vi "File_name_to_number.vi"(10 "Folder Path":path) -> (0 "Base File Name":string, 1 "Last file number":i32, 2 "File number =  file name?":bool, 3 "All Files in Dir":path[](array[path]))   [LabVIEW 2016]
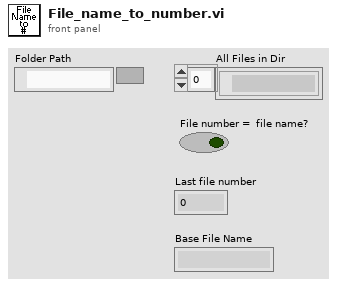
[diagram p1: front panel]
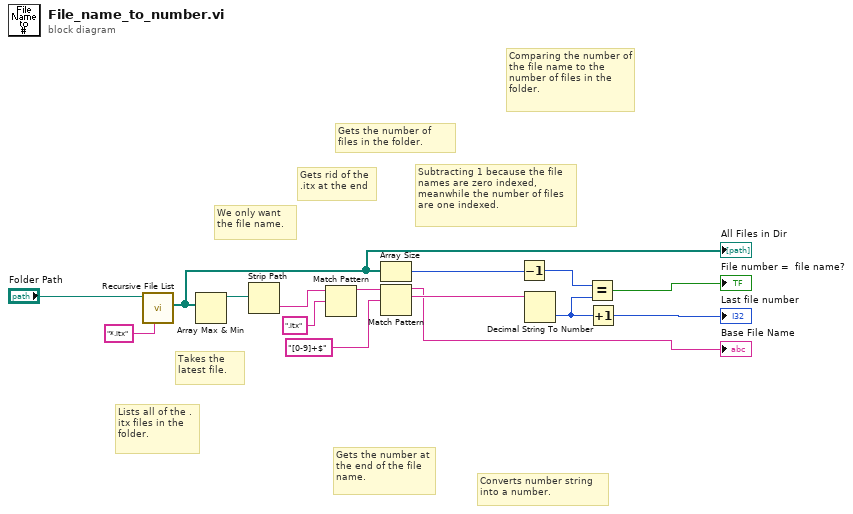
[diagram p0: block diagram]
diagram:
  # "Comparing the number of the file name to the number of files in the folder."
  # "Subtracting 1 because the file names are zero indexed, meanwhile the number of files are one indexed."
  # "Converts number string into a number."
  # "Gets the number at the end of the file name."
  # "Gets the number of files in the folder."
  # "Gets rid of the .itx at the end"
  # "We only want the file name."
  # "Takes the latest file."
  # "Lists all of the .itx files in the folder."
  n1 = call <vilib>:"Recursive File List.vi"("pattern"="*.itx", "Folder Path"="Folder Path") -> ("All Files in Dir"=w15:path[])  [unwired: 5 in, 4 out]
  "All Files in Dir" <- w15
  n2 = Array Max & Min(array=w15) -> (max value=w3:path)  [unwired: 3 out]
  n3 = Strip Path(path=w3) -> (name=w4:string)  [unwired: 1 out]
  n4 = Match Pattern(string=w4, regular expression=".itx") -> (before substring=w6:string)  [unwired: 1 in, 3 out]
  n5 = Array Size(array=w15) -> (size(s)=w9:i32)
  n6 = Match Pattern(string=w6, regular expression="[0-9]+$") -> (before substring=→"Base File Name":string, match substring=w14:string)  [unwired: 1 in, 2 out]
  n7 = Decrement(x=w9) -> (x-1=w10:i32)
  n8 = Decimal String To Number(string=w14) -> (number=w12:i32)  [unwired: 2 in, 1 out]
  n9 = Equal?(x=w10, y=w12) -> (x = y?=→"File number =  file name?":bool)
  n10 = Increment(x=w12) -> (x+1=→"Last file number":i32)
